vi "Read.vi"(8 "error in (no error)":errorcluster, 11 "Feeder Actor.lvlib:Solenoid.lvclass":refnum<class "Solenoid.lvclass">) -> (0 "error out":errorcluster, 3 "Feeder Actor.lvlib:Solenoid.lvclass 2":refnum<class "Solenoid.lvclass">)   [LabVIEW 2018, in "Feeder Actor.lvlib" / "Solenoid.lvclass"]
uses:
  Solenoid.lvclass
  Solenoid.lvclass/Solenoid.ctl
  <vilib>/DAQmx/read.llb/DAQmx Read (Digital Bool 1Line 1Point).vi
  <vilib>/DAQmx/miscellaneous.llb/DAQmx Fill In Error Info.vi
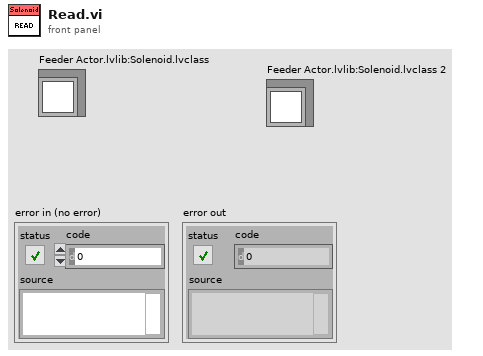
[diagram p1: front panel]
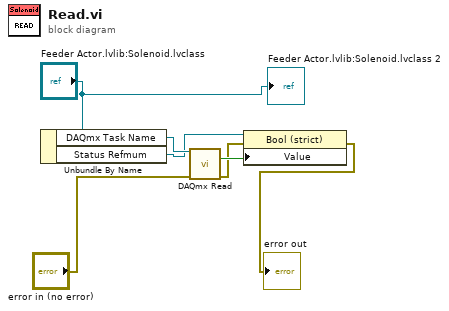
[diagram p0: block diagram]
diagram:
  n1 = Unbundle By Name("Feeder Actor.lvlib:Solenoid.lvclass") -> ("DAQmx Task Name"=w7:refnum<k21>, "Status Refmum"=w6:refnum<vi>)
  n2 = call-poly <vilib>:"DAQmx Read.vi"("task/channels in"=w7, "error in"="error in (no error)") -> ("data"=w5:bool, "error out"=w3:errorcluster)  [unwired: 11 in, 1 out]
  n3 = property class="Bool (strict)"(reference=w6, error in=w3, "Value"=w5) -> (error out=→"error out":errorcluster)  [unwired: 1 out]
  "Feeder Actor.lvlib:Solenoid.lvclass 2" <- "Feeder Actor.lvlib:Solenoid.lvclass"
